vi "Validate if event is selected.vi"(11 "Tree Selection":string) -> (0 "Selection type":T1)   [LabVIEW 2019, in "Panther Dashboard.lvlib"]
uses:
  Panther Dashboard.lvlib
  Selection Type--enum.ctl
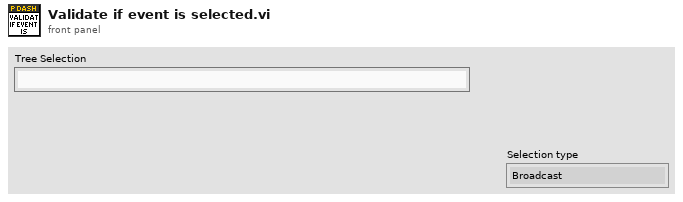
[diagram p1: front panel]
types:
  T1 = typedef "Panther Dashboard.lvlib/Selection Type--enum.ctl" = enum16{"Broadcast", "Request", "Module", "Public API"}
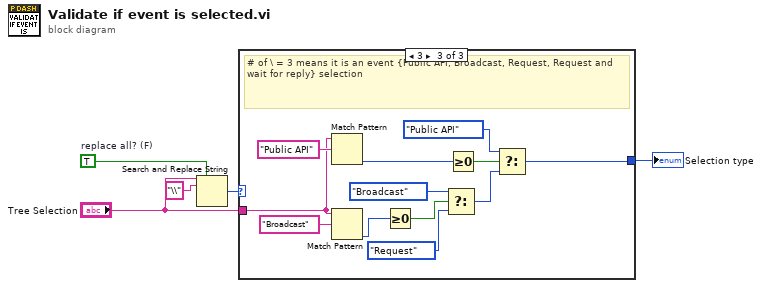
[diagram p0: block diagram]
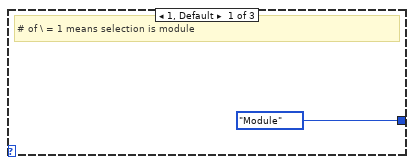
[diagram p2: hidden frame]
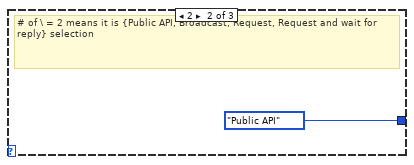
[diagram p3: hidden frame]
diagram:
  w4 = TRUE  # replace all? (F)
  n1 = Search and Replace String(replace all?=w4, input string="Tree Selection", search string="\\") -> (number of replacements=w3:i32)  [unwired: 5 in, 3 out]
  n2 = case shown="3" w3 {
    tunnel: [Selection_Type--enum."Module" Selection_Type--enum."Public API" w15] -> w1
    tunnel: "Tree Selection" -> [_ _ w13]
    frame 1, Default {
      # "# of \\ = 1 means selection is module"
    }
    frame 2 {
      # "# of \\ = 2 means it is {Public API, Broadcast, Request, Request and wait for reply} selection"
    }
    frame 3 {
      # "# of \\ = 3 means it is an event {Public API, Broadcast, Request, Request and wait for reply} selection"
      n3 = Match Pattern(string=w13, regular expression="Public API") -> (offset past match=w18:i32)  [unwired: 1 in, 3 out]
      n4 = Match Pattern(string=w13, regular expression="Broadcast") -> (offset past match=w12:i32)  [unwired: 1 in, 3 out]
      n5 = Greater Or Equal To 0?(x=w12) -> (x >= 0?=w11:bool)
      n6 = Select(t=Selection_Type--enum."Broadcast", s=w11, f=Selection_Type--enum."Request") -> (s? t:f=w8:T1)
      n7 = Greater Or Equal To 0?(x=w18) -> (x >= 0?=w17:bool)
      n8 = Select(t=Selection_Type--enum."Public API", s=w17, f=w8) -> (s? t:f=w15:T1)
    }
  }
  "Selection type" <- w1
